vi "1A Read Compass.vi"(11 "Reads a string\nfrom FPGA":string) -> (1 "Read string":string, 2 "heading":dbl, 3 "Result string":string)   [LabVIEW 2011]
doc: "Given a string from the compass, this vi will return the heading as a double\n\nThe given string must be in the digital compass format for NMEA 0183 - $HCHDH,180.0,,,,*F3,\\r\\n (or something close to that)\n\nThat string is taken from the compass' serial port"
uses:
  2-Think/2 Globals/2 Global.vi
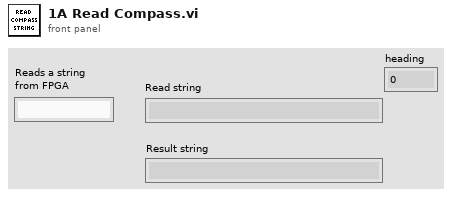
[diagram p1: front panel]
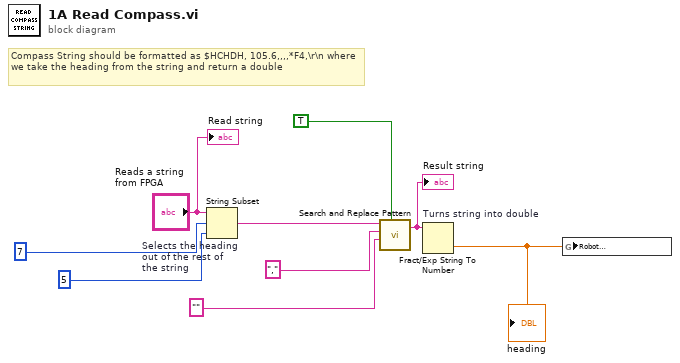
[diagram p0: block diagram]
diagram:
  # "Compass String should be formatted as $HCHDH, 105.6,,,,*F4,\\r\\n where we take the heading from the string and return a double"
  n1 = String Subset "Selects the heading\nout of the rest of\nthe string"(string="Reads a string\nfrom FPGA", offset (0)=7, length (rest)=5 ("length (rest)")) -> (substring=w7:string)
  n2 = call <vilib>:"Search and Replace Pattern.vi"("string"=w7, "regular expression (\"\")"="," ("regular expression (\"\")"), "replace string (\"\")"="" ("replace string (\"\")"), "replace all? (F)"=TRUE) -> ("result string"=w9:string)  [unwired: 1 in, 1 out]
  "Result string" <- w9
  n3 = Fract/Exp String To Number "Turns string into double"(string=w9) -> (number=w1:dbl)  [unwired: 3 in, 1 out]
  "heading" <- w1
  n4 = global write "2 Global.vi" "Robot\nHeading"(w1) -> ()
  "Read string" <- "Reads a string\nfrom FPGA"
